vi "Write Card Number From Control.vi"(8 "error in (no error)":errorcluster, 10 "Card Number":dbl format="%#_13g", 11 "Display Panel.lvlib:Display Panel V3.lvclass":refnum<class "Display Panel V3.lvclass">) -> (0 "error out":errorcluster, 3 "reference out":refnum<class "Display Panel V3.lvclass">)   [LabVIEW 2016, in "Display Panel.lvlib" / "Display Panel V3.lvclass"]
uses:
  Display Panel V3.lvclass
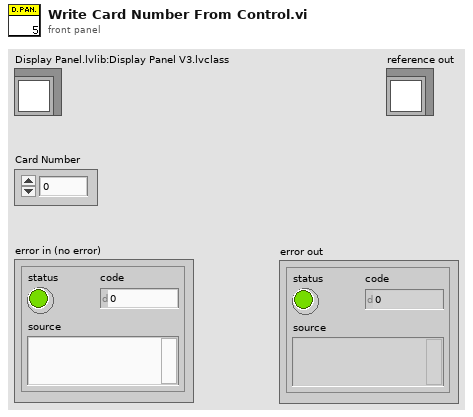
[diagram p1: front panel]
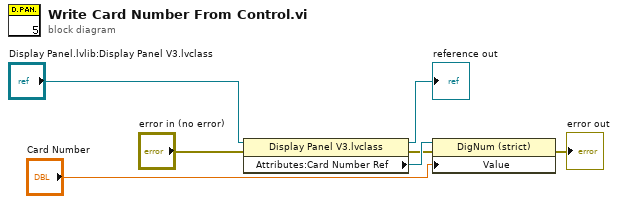
[diagram p0: block diagram]
diagram:
  n1 = property class="Display Panel V3.lvclass"(reference="Display Panel.lvlib:Display Panel V3.lvclass", error in="error in (no error)") -> (reference out=→"reference out":refnum<class "Display Panel V3.lvclass">, error out=w4:errorcluster, "Attributes:Card Number Ref"=w6:refnum<vi>)
  n2 = property class="DigNum (strict)"(reference=w6, error in=w4, "Value"="Card Number") -> (error out=→"error out":errorcluster)  [unwired: 1 out]
